vi "GetVoltNumber.vi"(0 "BMUNO":u32=10, 1 "类型":u32(ring)=4 items=["PCI5121"=1, "PCI9810"=2, "USBCAN1"=3, "USBCAN2"=4, "PCI9820"=5, "CAN232"=6, "PCI5110"=7, "CANLite(mini)"=8, "ISA9620"=9, "ISA5420"=10, "PC104CAN"=11, "CANET"=17, "DNP9810"=13, "USBCAN-E-U"=20, "USBCAN-2E-U"=21], 2 "设备索引":u32(ring) items=["0", "1", "2", "3", "4", "5", "6", "7", "8", "9", "10", "11", "12", "13", "14", "15", ""], 3 "CAN路数":u32(ring) items=["0", "1"], 11 "time out":u32) -> (4 "recv ok?":bool, 6 "Value":u64)   [LabVIEW 2013]
uses:
  AutoBurn/Settings/ControlCAN.dll
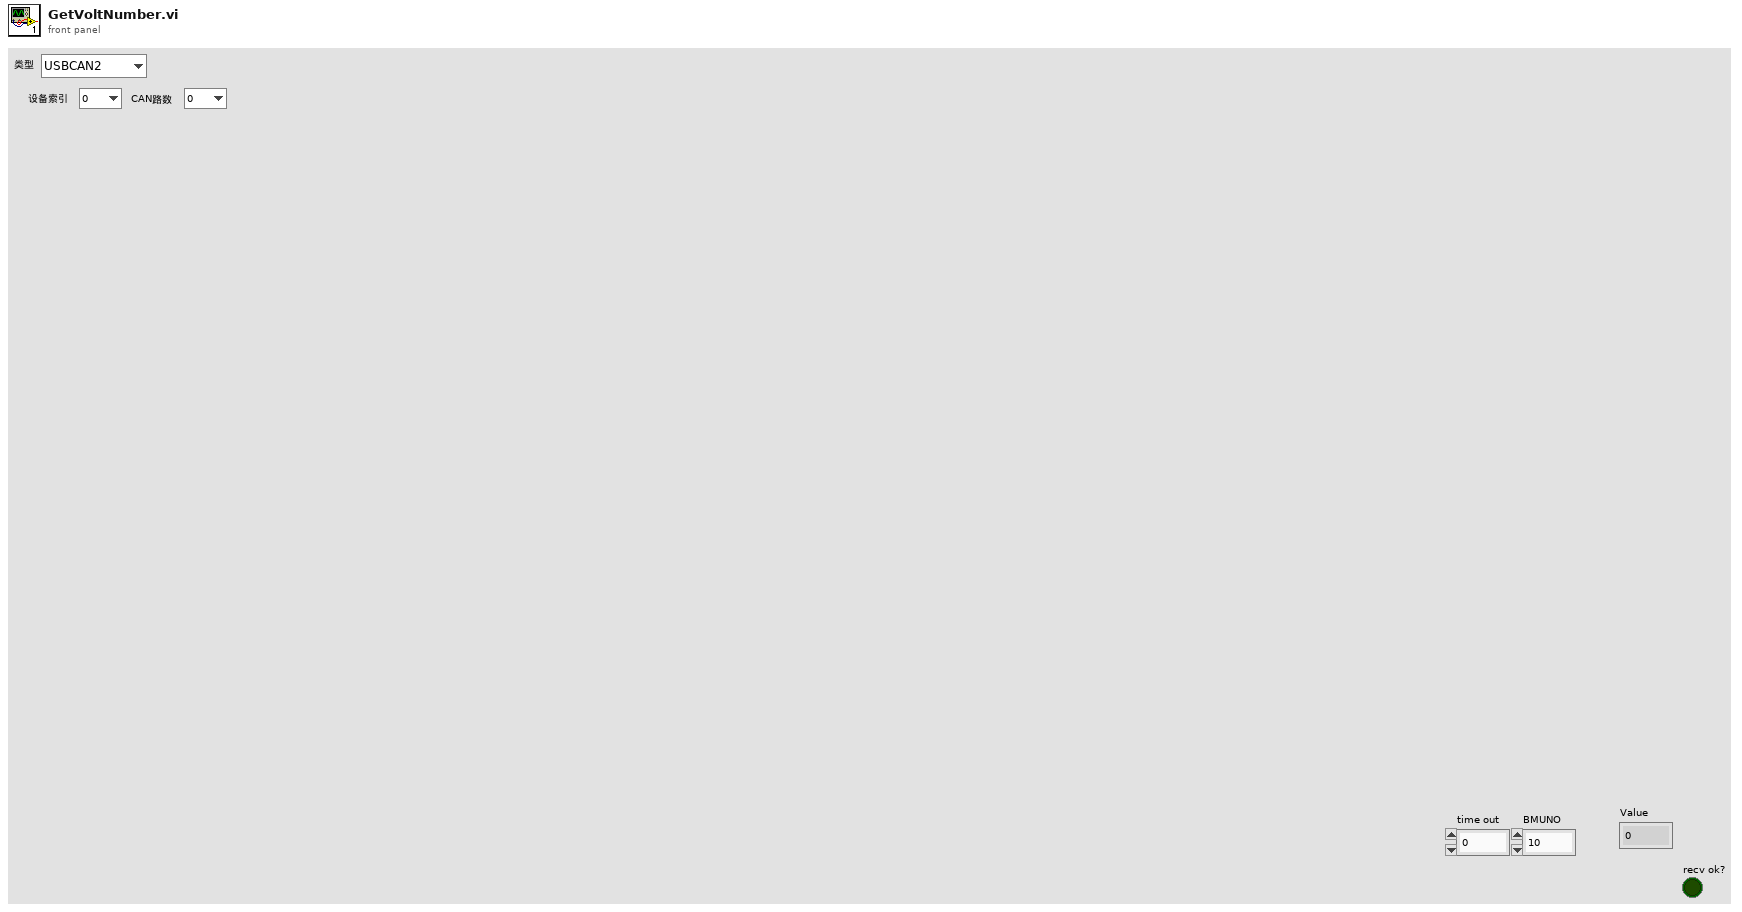
[diagram p1: front panel]
types:
  T1 = cluster{"ID":u32, "TimeStamp":u32, "TimeFlag":u8, "SendType":u8, "RemoteFlag":u8, "ExternFlag":u8, "DataLen":u8, u8, u8, u8, u8, u8, u8, u8, u8, u8, u8, u8}
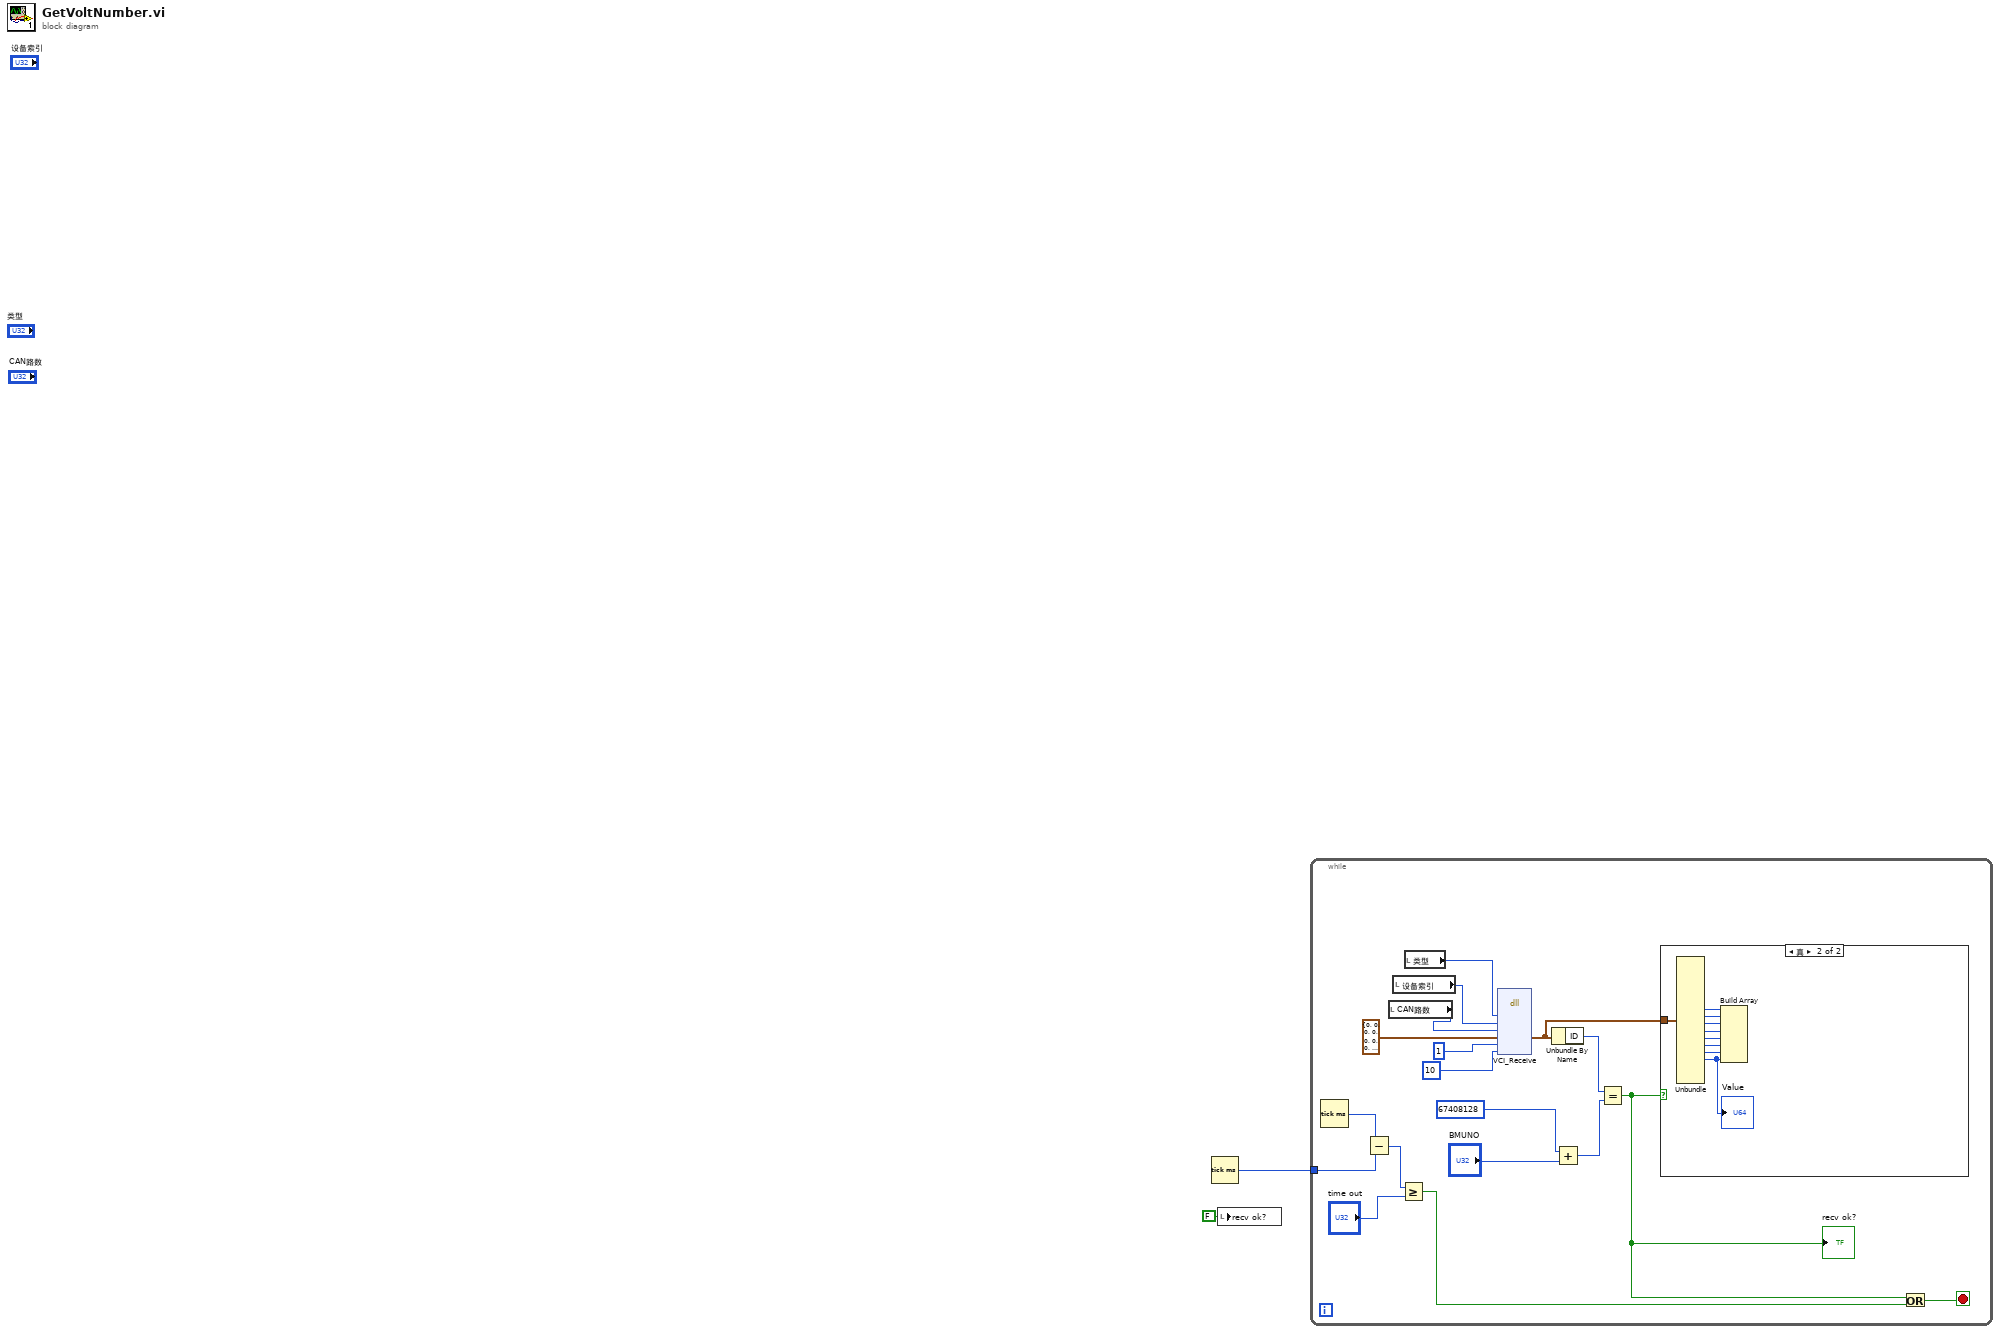
[diagram p0: block diagram]
diagram:
  n1 = Tick Count (ms)() -> (millisecond timer value=w2:u32)
  n2 = local write "recv ok?"(FALSE ("x = y?")) -> ()
  n3 = while {
    tunnel: w2 -> [w13]
    stop <- w7 stop-if-true
    n4 = Tick Count (ms)() -> (millisecond timer value=w14:u32)
    n5 = Subtract(x=w14, y=w13) -> (x-y=w12:u32)
    n6 = local read "CAN路数"() -> (w18:u32)
    n7 = local read "设备索引"() -> (w15:u32)
    n8 = Greater Or Equal?(x=w12, y="time out") -> (x >= y?=w8:bool)
    n9 = local read "类型"() -> (w16:u32)
    n10 = dll-call lib="F:/Bluewave New Energy/SVN_Work/AutoTest_TestStand/trunk/AutoTest_TestStand/Driver/ZlgCan/BHN01/AutoBurn/Settings/ControlCAN.dll" fn="VCI_Receive"("DeviceType"=w16, "DeviceInd"=w15, "CANInd"=w18, "pReceive"=T1 {"ID"=0, "TimeStamp"=0, "TimeFlag"=0, "SendType"=0, "RemoteFlag"=0, "ExternFlag"=0, "DataLen"=0, 0, 0, 0, 0, 0, 0, 0, 0, 0, 0, 0}, "Len"=u32 1, "WaitTime"=10) -> ("pReceive"=w6:T1)  [unwired: 8 in, 3 out]
    n11 = Unbundle By Name(w6) -> ("ID"=w10:u32)
    n12 = Add(x=u32 67408128, y="BMUNO") -> (x+y=w3:u32)
    n13 = Equal?(x=w10, y=w3) -> (x = y?=w9:bool)
    "recv ok?" <- w9
    n14 = case shown="真" w9 {
      tunnel: w6 -> [_ w29]
      frame False {
      }
      frame True {
        n15 = Unbundle(w29) -> (w28:u8, w27:u8, w26:u8, w25:u8, w24:u8, w23:u8, w22:u8, w21:u8)  [unwired: 10 out]
        "Value" <- w21
        n16 = Build Array(w28, w27, w26, w25, w24, w23, w22, w21) -> ()  [unwired: 1 out]
      }
    }
    n17 = Or(x=w9, y=w8) -> (x .or. y?=w7:bool)
  }
